vi "Set Value Table.vi"(8 "error in (no error)":errorcluster, 9 "XNET Signal":refnum<k21>="ABSActive\nDatabase_FCA", 11 "Channel Ref in":T1 format="%.0x") -> (0 "error out":errorcluster)   [LabVIEW 2018, in "CAN Gateway System Explorer.lvlib"]
uses:
  CAN Gateway System Explorer.lvlib
  <vilib>/NI Veristand/Custom Device API/Custom Device Item Ref.ctl
  <vilib>/xnet/xnet.llb/XNET Get DBC Mode.ctl
  <vilib>/xnet/xnet.llb/XNET Database Get DBC Attribute (Signal).vi
  <vilib>/NI Veristand/Custom Device API/Custom Device API.lvlib
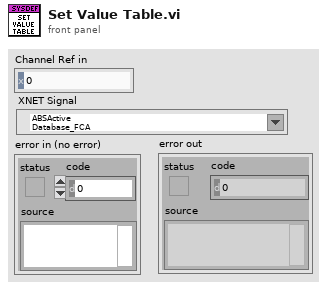
[diagram p1: front panel]
types:
  T1 = typedef "Custom Device API.lvlib/Custom Device Item Ref.ctl" = u64
  T2 = typedef "XNET Get DBC Mode.ctl" = u32
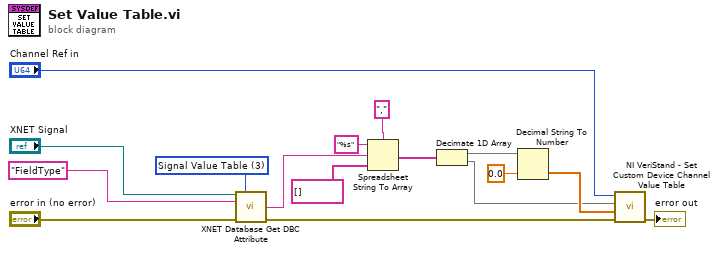
[diagram p0: block diagram]
diagram:
  w15 = T2 3 items=["Attribute Value", "Enumeration", "Attribute Name List", "Signal Value Table"] ("mode")
  n1 = call-poly <vilib>:"XNET Database Get DBC Attribute.vi"("signal in"="XNET Signal", "mode"=w15, "attribute name"="FieldType", "error in (no error)"="error in (no error)") -> ("attribute text"=w13:string, "error out"=w3:errorcluster)  [unwired: 8 in, 2 out]
  n2 = Spreadsheet String To Array(delimiter (Tab)=",", format string="%s", spreadsheet string=w13, array type (2D Dbl)=string[] []) -> (array=w10:string[])
  n3 = Decimate 1D Array(w10) -> (w6:string[], w1:string[])
  n4 = Decimal String To Number(string=w6, default (0L)=0.0) -> (number=w7:dbl[])  [unwired: 1 in, 1 out]
  n5 = call <vilib>:"NI VeriStand - Set Custom Device Channel Value Table.vi"("error in (no error)"=w3, "Values"=w7, "Names"=w1, "Channel Ref in"="Channel Ref in") -> ("error out"=→"error out":errorcluster)  [unwired: 6 in, 1 out]
